vi "Onset detection.vi"(9 "Pre-onset ms (50)":dbl=50.0, 10 "dt":dbl, 11 "Data":dbl[](graph)) -> (0 "onset threshold":dbl, 1 "Cursor X":dbl, 2 "Onset index":i32, 3 "Data out":dbl[](graph))   [LabVIEW 2016]
uses:
  <vilib>/Analysis/NI_AALPro.lvlib
  <vilib>/Analysis/NI_AALBase.lvlib
panel:
  out "Data":cluster{"Time":dbl[], "Data":dbl[]}[](graph)
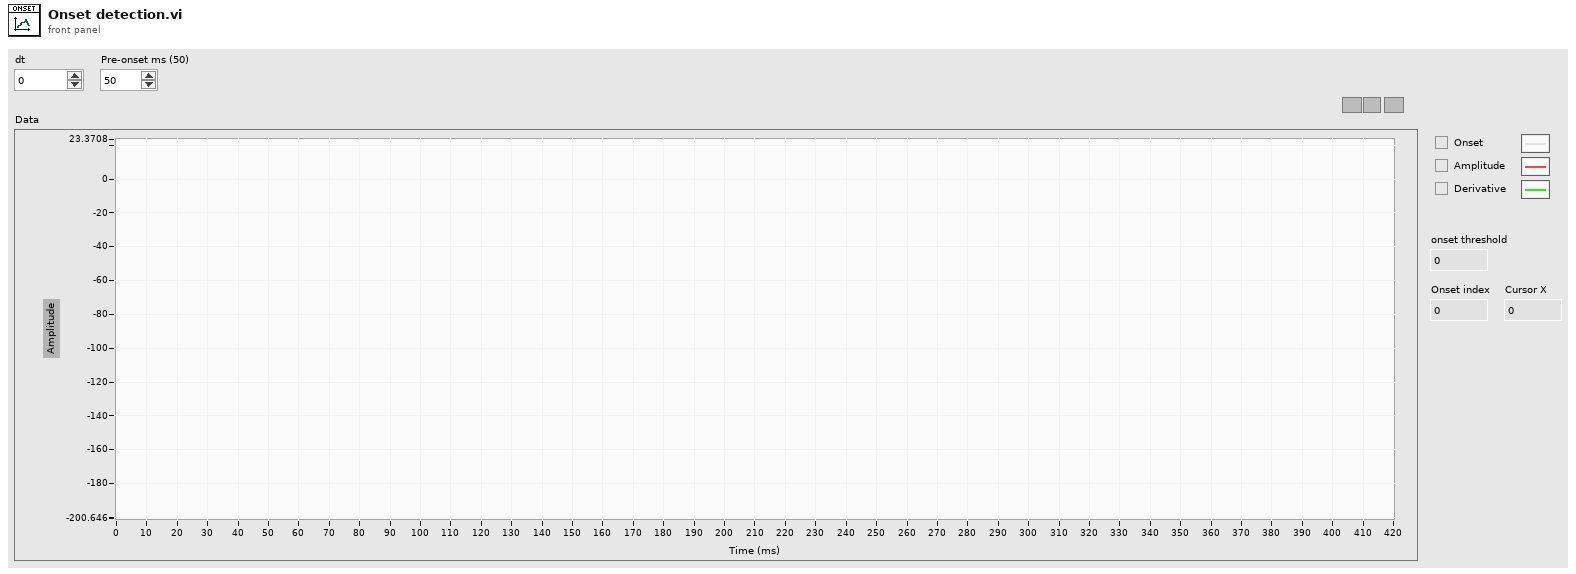
[diagram p1: front panel]
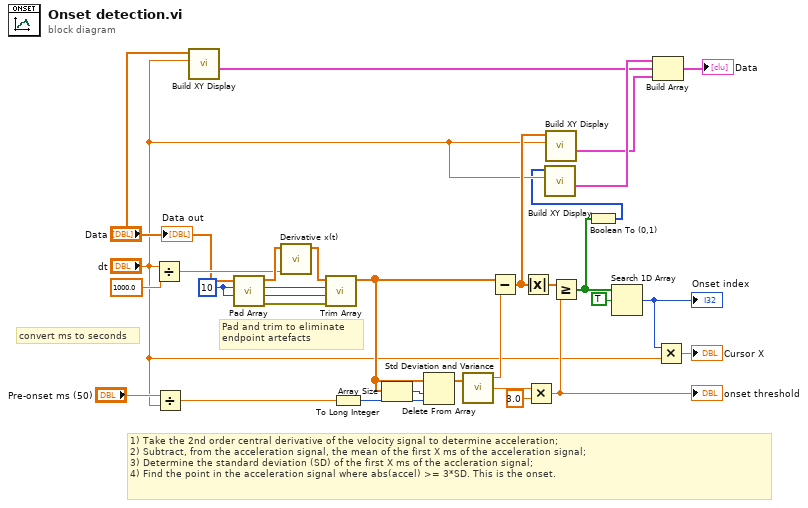
[diagram p0: block diagram]
diagram:
  w30 = 10 ("pre")
  # "Pad and trim to eliminate endpoint artefacts"
  # "convert ms to seconds"
  # "1) Take the 2nd order central derivative of the velocity signal to determine acceleration;\n2) Subtract, from the acceleration signal, the mean of the first X ms of the acceleration signal;\n3) Determine the standard deviation (SD) of the first X ms of the accleration signal;\n4) Find the point in the acceleration signal where abs(accel) >= 3*SD. This is the onset."
  n1 = Divide(x="dt", y=1000.0) -> (x/y=w24:dbl)
  n2 = Divide(x="Pre-onset ms (50)", y="dt") -> (x/y=w20:dbl)
  n3 = call <userlib>:"Build XY Display.vi"("dt"="dt", "Data"="Data") -> ("Data"=w2:cluster{"Time":dbl[], "Data":dbl[]})  [unwired: 6 in, 3 out]
  n4 = call <userlib>:"Pad Array.vi"("post"=w30, "pre"=w30, "Array"="Data") -> ("error out"=w29:errorcluster, "post"=w16:i32, "pre"=w17:i32, "Padded array"=w31:dbl[])  [unwired: 5 in]
  n5 = call <vilib>:"Derivative x(t).vi"("dt"=w24, "X"=w31) -> ("dX/dt"=w18:dbl[])  [unwired: 8 in, 1 out]
  n6 = call <userlib>:"Trim Array.vi"("error in"=w29, "post"=w16, "pre"=w17, "Array"=w18) -> ("Trimmed array"=w15:dbl[])  [unwired: 6 in, 1 out]
  n7 = To Long Integer(number=w20) -> (32bit integer=w19:i32)
  n8 = Array Size(array=w15) -> (size(s)=w21:i32)
  n9 = Delete From Array(array=w15, length=w21, index=w19) -> (array with subset deleted=w10:dbl[])  [unwired: 1 out]
  n10 = call <vilib>:"Std Deviation and Variance.vi"("X"=w10) -> ("mean"=w9:dbl, "standard deviation"=w13:dbl)  [unwired: 1 in, 1 out]
  n11 = Subtract(x=w15, y=w9) -> (x-y=w7:dbl[])
  n12 = Absolute Value(x=w7) -> (abs(x)=w28:dbl[])
  n13 = Multiply(x=w13, y=3.0) -> (x*y=w11:dbl)
  "onset threshold" <- w11
  n14 = call <userlib>:"Build XY Display.vi"("dt"="dt", "Data"=w7) -> ("Data"=w3:cluster{"Time":dbl[], "Data":dbl[]})  [unwired: 6 in, 3 out]
  n15 = Greater Or Equal?(x=w28, y=w11) -> (x >= y?=w27:bool[])
  n16 = Boolean To (0,1)(Boolean=w27) -> (0, 1=w5:i16[])
  n17 = call <userlib>:"Build XY Display.vi"("dt"="dt", "Data"=w5) -> ("Data"=w4:cluster{"Time":dbl[], "Data":dbl[]})  [unwired: 6 in, 3 out]
  n18 = Search 1D Array(1D array=w27, element=TRUE) -> (index of element=w14:i32)  [unwired: 1 in]
  "Onset index" <- w14
  n19 = Build Array(w4, w2, w3) -> (→"Data":cluster{"Time":dbl[], "Data":dbl[]}[])
  n20 = Multiply(x=w14, y="dt") -> (x*y=→"Cursor X":dbl)
  "Data out" <- "Data"
